vi "Set Menu Item Name.vi"(7 "item tag":string, 8 "error in (no error)":errorcluster, 10 "item name":string, 11 "Menu in":refnum<class "Menu.lvclass">) -> (0 "error out":errorcluster, 3 "Menu out":refnum<class "Menu.lvclass">)   [LabVIEW 2021, in "Menu.lvlib" / "Menu.lvclass"]
uses:
  Menu.lvclass
  Menu.lvclass/Menu.ctl
  <vilib>/Utility/miscctls.llb/LVMapReplaceAction.ctl
  MenuItems.ctl
  <vilib>/Utility/miscctls.llb/LVMenuShortCut.ctl
  Picture2D/src/2DPictureControl/2DPictureControl.lvclass
  Picture2D/src/Picture/Image.lvclass
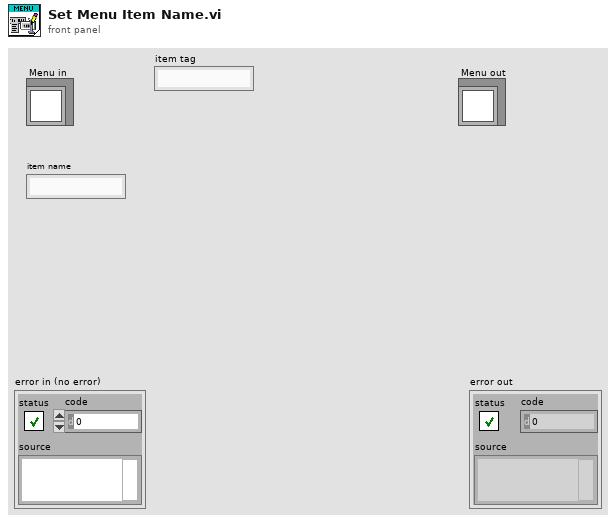
[diagram p1: front panel]
types:
  T1 = typedef "Menu.lvlib/Menu.lvclass/MenuItems.ctl" = cluster{"Item Name":string, "Short Cut":T2, "Checked":bool, "Enable":bool, "After item":string, "Item Tags":string[], "Item Names":string[], "Picture":refnum<class "Image.lvclass">, "Hilite Picture":refnum<class "Image.lvclass">, "Displayed":bool}
  T2 = typedef "LVMenuShortCut.ctl" = cluster{"Include Shift Key?":bool, "Include Ctrl Key?":bool, "Shortcut Key":string}
  T3 = typedef "LVMapReplaceAction.ctl" = enum32{"Modify Entry only if found", "Add or Modify Entry", "Delete Entry"}
  T4 = typedef "Menu.lvlib/Menu.lvclass/Data.ctl" = cluster{"MenuMap":map{string, T1}, "PictRef":refnum<vi>, "MenuSelectionEvent":refnum<user-event>, "TopMenuSpacing":i32, "MenuSpacing":i32, "CloseEvent":refnum<user-event>, "TR_ManageMenuRef":refnum<vi>, "MenuColors":T5, "RTMPath":path, "RTMVIReference":refnum<vi>, "RTMMenuReference":refnum<k9>, "CtlRef":refnum<vi>, "User-Specified Font":refnum<class "Font.lvclass">, "Desired Font":enum16{"User-specified Font", "Application Font", "System Font", "Dialog Font"}, "SubMenuIcon":T6, "SubMenuIconClosed":refnum<class "Picture2D.lvclass">, "SubMenuIconOpened":refnum<class "Picture2D.lvclass">}
  T5 = typedef "Menu.lvlib/Menu.lvclass/MenuColors.ctl" = cluster{"Text":refnum<class "Color.lvclass">, "HiliteText":refnum<class "Color.lvclass">, "Background":refnum<class "Color.lvclass">, "BorderColor":refnum<class "Color.lvclass">, "Hilite":refnum<class "Color.lvclass">}
  T6 = typedef "Menu.lvlib/Menu.lvclass/SubMenuIcon.ctl" = enum16{"LabVIEW", "Windows", "Custom"}
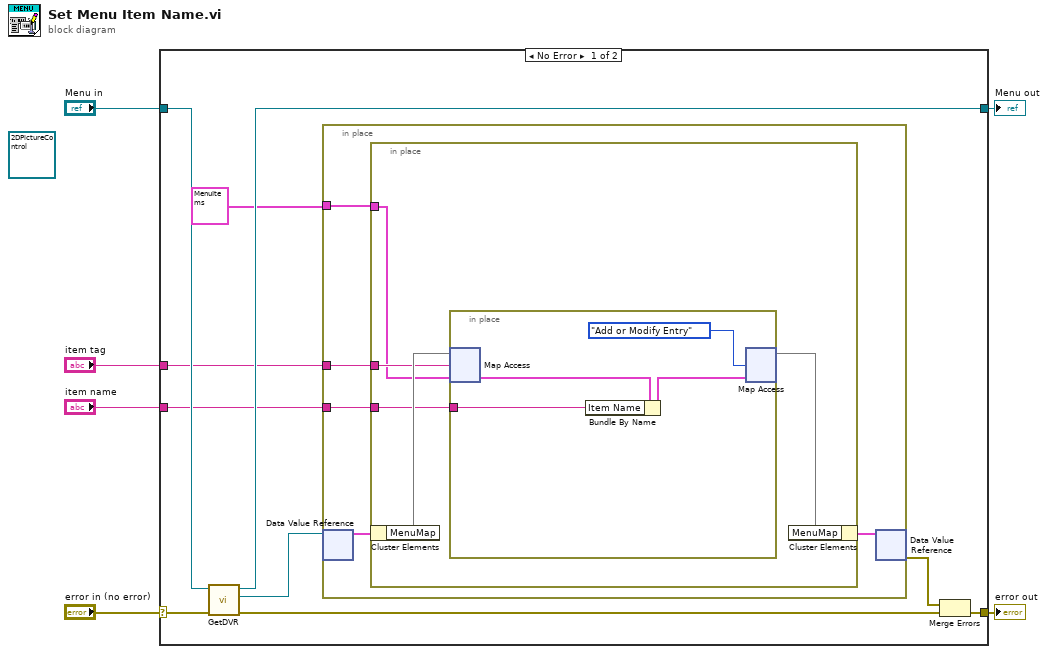
[diagram p0: block diagram]
diagram:
  (unwired) refnum<class "2DPictureControl.lvclass"> refnum ("Picture")
  (unwired) refnum<class "2DPictureControl.lvclass"> refnum ("Picture")
  n1 = case shown="No Error" "error in (no error)" {
    selector: "error in (no error)" -> [w16 w32]
    tunnel: [w8 w32] -> w5
    tunnel: [w14 w31] -> w3
    tunnel: "Menu in" -> [w13 w31]
    tunnel: "item name" -> [w10 _]
    tunnel: "item tag" -> [w11 _]
    frame No Error {
      n2 = call "GetDVR.vi"("error in (no error)"=w16, "Menu in"=w13) -> ("error out"=w15:errorcluster, "DVR"=w12:refnum<data-value>, "Menu out"=w14:refnum<class "Menu.lvclass">)  [unwired: 7 in]
      n3 = in-place {
        in-place-border: w11 -> [w20]
        in-place-border: w10 -> [w18]
        in-place-border: T1 {"Item Name"="", "Short Cut"={"Include Shift Key?"=FALSE, "Include Ctrl Key?"=FALSE, "Shortcut Key"=""}, "Checked"=FALSE, "Enable"=FALSE, "After item"="", "Item Tags"=[], "Item Names"=[], "Picture"=refnum, "Hilite Picture"=refnum, "Displayed"=FALSE} ("Menu") -> [w17]
        n4 = in-place-dvr #1(w12) -> (w21:T4)  [unwired: 1 out]
        n5 = in-place {
          in-place-border: w20 -> [w25]
          in-place-border: w18 -> [w23]
          in-place-border: w17 -> [w22]
          n6 = in-place-cluster #2(w21) -> ("MenuMap"=w26:map{string, T1})
          n7 = in-place {
            in-place-border: w23 -> [w29]
            n8 = in-place-map #3(w26, w25, w22) -> (w28:T1)  [unwired: 1 out]
            n9 = Bundle By Name(cluster=w28, "Item Name"=w29) -> (w27:T1)
            n10 = in-place-map #3(w27, LVMapReplaceAction."Add or Modify Entry" ("action")) -> (w24:map{string, T1})  [unwired: 2 out]
          }
          n11 = in-place-cluster #2("MenuMap"=w24) -> (w19:T4)
        }
        n12 = in-place-dvr #1(w19) -> (w7:errorcluster)  [unwired: 1 out]
      }
      n13 = Merge Errors(w7, w15) -> (w8:errorcluster)
    }
    frame Error {
    }
  }
  "error out" <- w5
  "Menu out" <- w3
